vi "Add Attribute at Index.vi"(4 "Insertion Index":i32=-1, 6 "Unique ID":string, 8 "error in (no error)":errorcluster, 11 "Linked List Definition in":refnum<class "Linked List Definition.lvclass">) -> (0 "error out":errorcluster, 3 "Linked List Definition out":refnum<class "Linked List Definition.lvclass">)   [LabVIEW 2020, in "Linked Lists.lvlib" / "Linked List Definition.lvclass"]
uses:
  <vilib>/gpm_packages/@cs/linked-list/Source/Linked List/Linked List Definition/Linked List Definition.lvclass
  <vilib>/gpm_packages/@cs/linked-list/Source/Linked List/Linked List Definition/Linked List Definition.lvclass/Linked List Definition.ctl
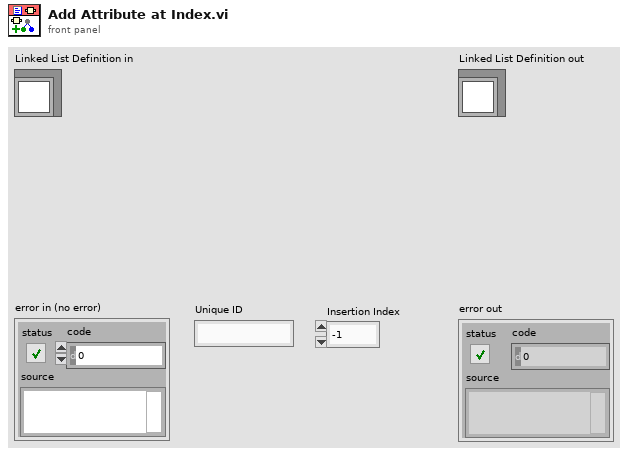
[diagram p1: front panel]
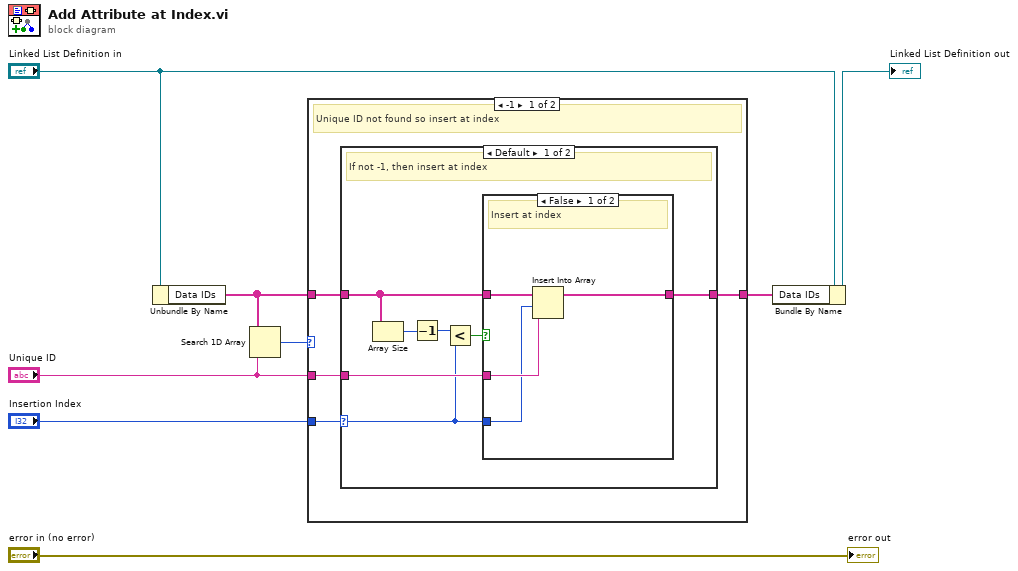
[diagram p0: block diagram]
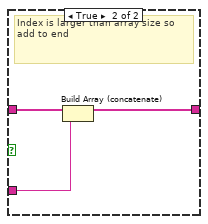
[diagram p2: hidden frame]
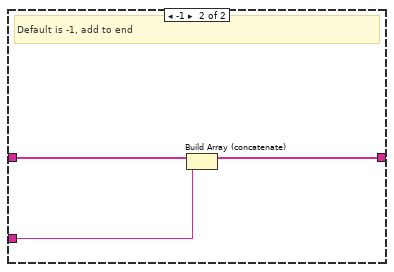
[diagram p3: hidden frame]
diagram:
  n1 = Unbundle By Name("Linked List Definition in") -> ("Data IDs"=w7:string[])
  n2 = Search 1D Array(1D array=w7, element="Unique ID") -> (index of element=w8:i32)  [unwired: 1 in]
  n3 = case shown="-1" w8 {
    tunnel: w7 -> [w12 w30]
    tunnel: "Unique ID" -> [w11 _]
    tunnel: [w10 w30] -> w2
    tunnel: "Insertion Index" -> [w9 _]
    frame -1 {
      # "Unique ID not found so insert at index"
      n4 = case shown="Default" w9 {
        selector: w9 -> [w13 _]
        tunnel: w12 -> [w15 w29]
        tunnel: w11 -> [w18 w28]
        tunnel: [w19 w27] -> w10
        frame Default {
          # "If not -1, then insert at index"
          n5 = Array Size(array=w15) -> (size(s)=w17:i32)
          n6 = Decrement(x=w17) -> (x-1=w16:i32)
          n7 = Less?(x=w16, y=w13) -> (x < y?=w14:bool)
          n8 = case shown="False" w14 {
            tunnel: [w23 w25] -> w19
            tunnel: w18 -> [w22 w24]
            tunnel: w15 -> [w21 w26]
            tunnel: w13 -> [w20 _]
            frame False {
              # "Insert at index"
              n9 = Insert Into Array(array=w21, index=w20, new element=w22) -> (w23:string[])
            }
            frame True {
              # "Index is larger than array size so add to end"
              n10 = Build Array (concatenate)(w26, w24) -> (w25:string[])
            }
          }
        }
        frame -1 {
          # "Default is -1, add to end"
          n11 = Build Array (concatenate)(w29, w28) -> (w27:string[])
        }
      }
    }
    frame Default {
      # "Unique ID already exists"
    }
  }
  n12 = Bundle By Name(cluster="Linked List Definition in", "Data IDs"=w2) -> (→"Linked List Definition out":refnum<class "Linked List Definition.lvclass">)
  "error out" <- "error in (no error)"
